vi "Get_Index_of_the_Tag.vi"(11 "Tag's name":string) -> (3 "Index of the Tag":i32)   [LabVIEW 2020, in "DriverCommon.lvlib"]
uses:
  DriverCommon.lvlib
  Load_TagServer.lvlib
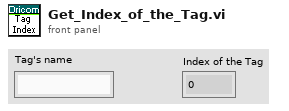
[diagram p1: front panel]
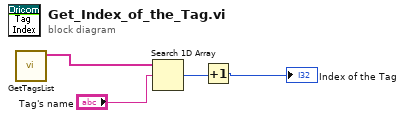
[diagram p0: block diagram]
diagram:
  n1 = call "GetTagsList.vi"() -> ("Tags"=w3:string[])  [unwired: 10 in, 1 out]
  n2 = Search 1D Array(1D array=w3, element="Tag's name") -> (index of element=w2:i32)  [unwired: 1 in]
  n3 = Increment(x=w2) -> (x+1=→"Index of the Tag":i32)
